vi "getIndex.vi"(11 "ModbusBuffer in":refnum<class "ModbusBufferBuilder.lvclass">) -> (2 "Index":i32, 3 "ModbusBuffer out":refnum<class "ModbusBufferBuilder.lvclass">)   [LabVIEW 2016, in "ModbusBufferBuilder.lvclass"]
uses:
  ModbusBufferBuilder.lvclass
  ModbusBufferBuilder.lvclass/ModbusBufferBuilder.ctl
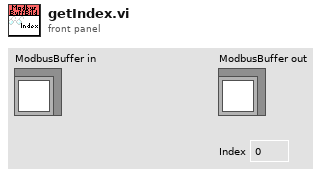
[diagram p1: front panel]
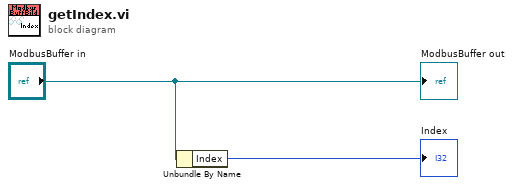
[diagram p0: block diagram]
diagram:
  n1 = Unbundle By Name("ModbusBuffer in") -> ("Index"=→"Index":i32)
  "ModbusBuffer out" <- "ModbusBuffer in"
